vi "Joy Processing.vi"() -> (5 "Plug in titles":string[](array[string]), 7 "Plug in values":string[](array[string]))   [LabVIEW 2021]
uses:
  Globals/Meas_global.vi
panel:
  out "XY Graph":T1(graph)
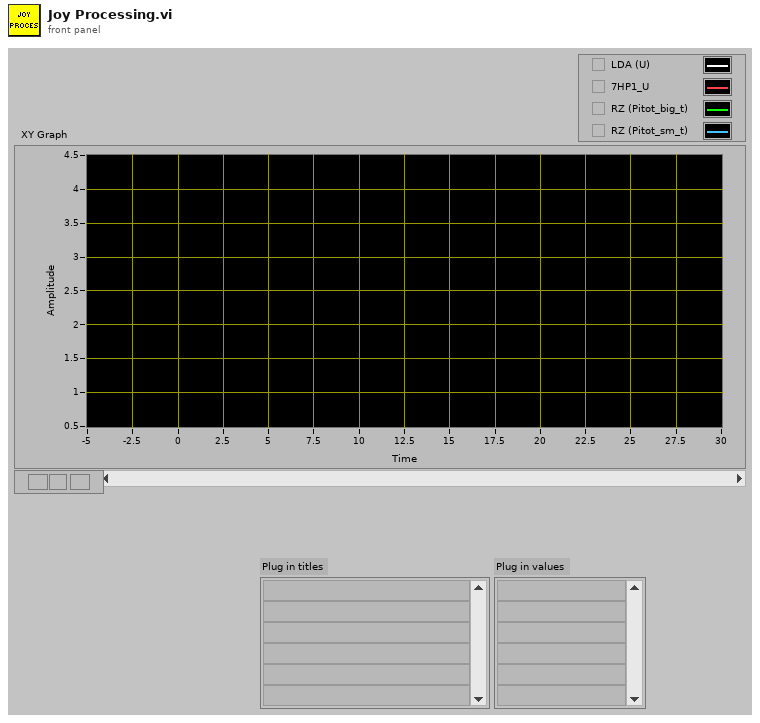
[diagram p1: front panel]
types:
  T1 = cluster{"Time (s)":dbl[], "Velocity (m/s)":dbl[]}[]
  T2 = typedef "Analysis_info_cluster.ctl" = cluster{"Colour":u32, "Inst type":T3, "Inst name":string, "Symbol":string, "Code name":string, "Extra Info":string, "Inst Array":T4, "Extra Titles":string[], "Extra Values":string[], "U":dbl, "u^2":dbl, "u^3":dbl, "u^4":dbl, "Skew_u":dbl, "Kurt_u":dbl, "Sd Error in Mean":dbl, "% u'/U":dbl, "X":dbl, "Y":dbl, "Z":dbl, "Timescale integral Estimate":dbl, "Sd Error in Variance":dbl, "Calib File":path, "Calib Constants":dbl[], "Output Position":bool, "Stats":enum16{"None", "Basic", "Full"}, "Av Sampling Rate":dbl, "Av No of Samples":dbl, "Total Meas Time (s)":dbl, "ADAM Ch Name":string, "Max value":dbl, "Min value":dbl, "Req Sample Rate Hz":dbl, "Sync Delay Time (s)":dbl, "Ch No":i16, "Device":string, "Use Latest Calib":bool, "Port":string, "Metadata Ch Names":string[], "Metadata Ch Values":string[], "Label":string}
  T3 = typedef "Inst_type.ctl" = enum16{"Raw voltage", "Raw with zero offsetting", "Propeller anemometer", "Pressure Transducer", "Pitot-static tube", "Hot wire", "Cross wire 1", "Cross wire 2", "Generic Linear", "Generic Polynomial", "Generic BackPoly", "Fast FID", "Thermocouple", "Cold wire", "Pulsed Wire", "LDA Vel", "LDA Tran time", "LDA Arr time", "Microphone"}
  T4 = typedef "Instrument_Array.ctl" = enum16{"PWA", "LDA", "Analogue"}
  T5 = typedef "Time_Trace_Cluster.ctl" = cluster{"Weighting":dbl[], "Voltage":dbl[], "Eng Values":dbl[]}
  T6 = cluster{"Time (s)":dbl[], "Velocity (m/s)":dbl[]}
  T7 = typedef "Correlation_cluster1.ctl" = cluster{"U inst":string, "uw":dbl, "u^2w":dbl, "uw^2":dbl, "uw/u'w'":dbl, "W inst":string, "uw^3":dbl, "u^3w":dbl, "u^2w^2":dbl, "Index U":i32, "Index W":i32, "Error info":string[], "Paired Sampling Rate (Hz)":dbl, "u^2 Paired":dbl, "w^2 Paired":dbl, "Time Window (ms)":dbl}
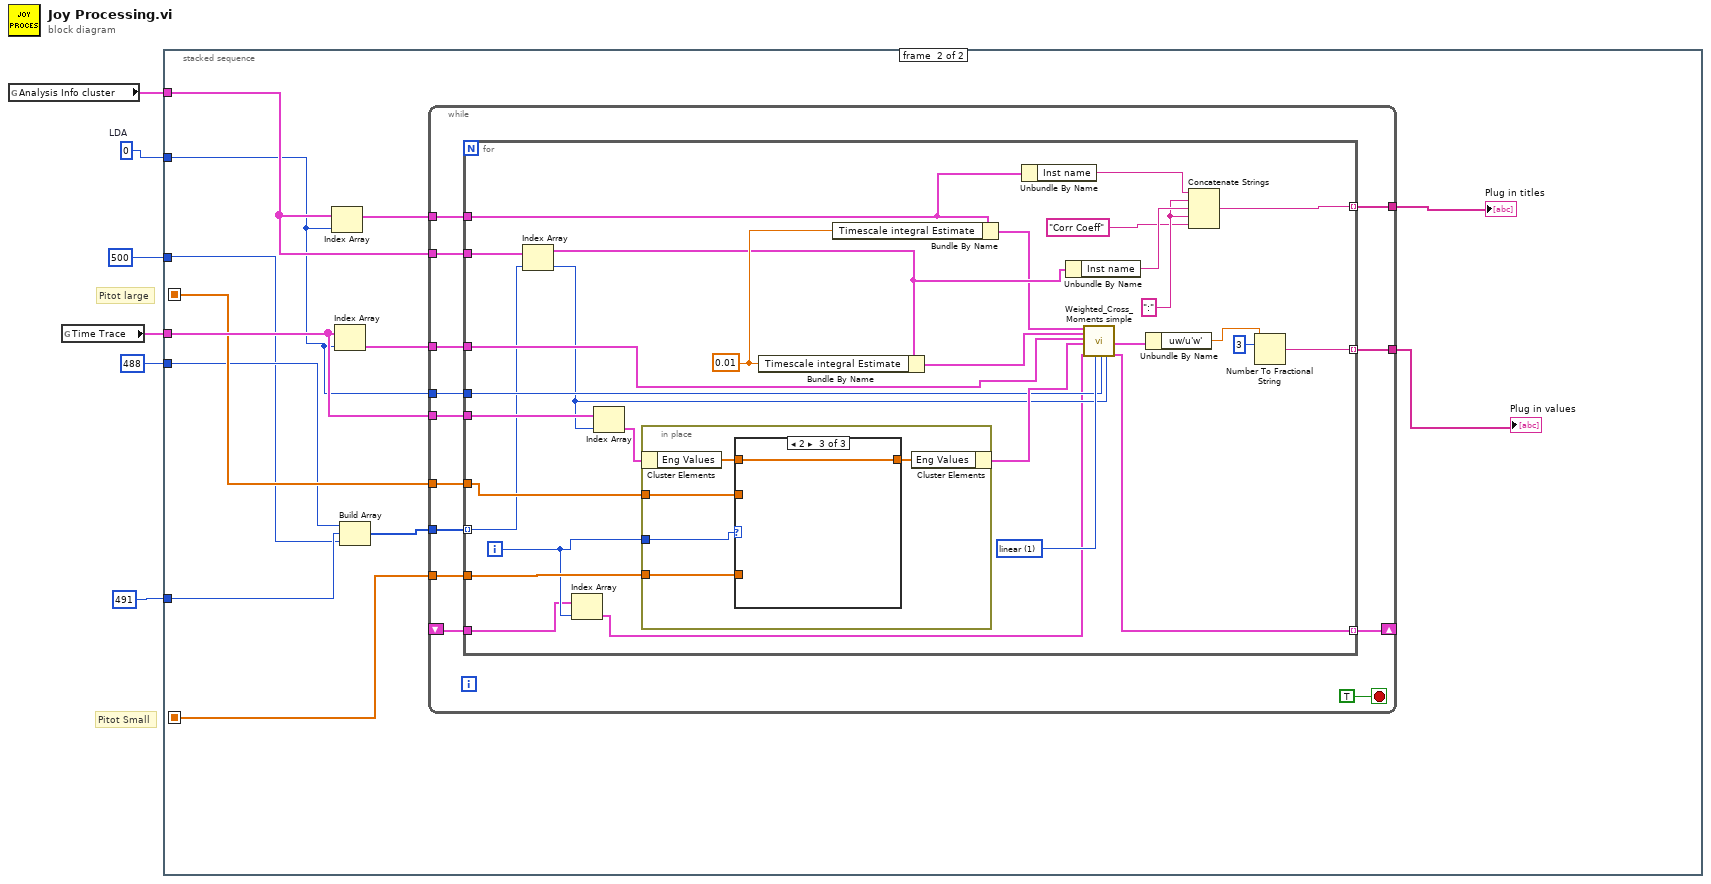
[diagram p0: block diagram]
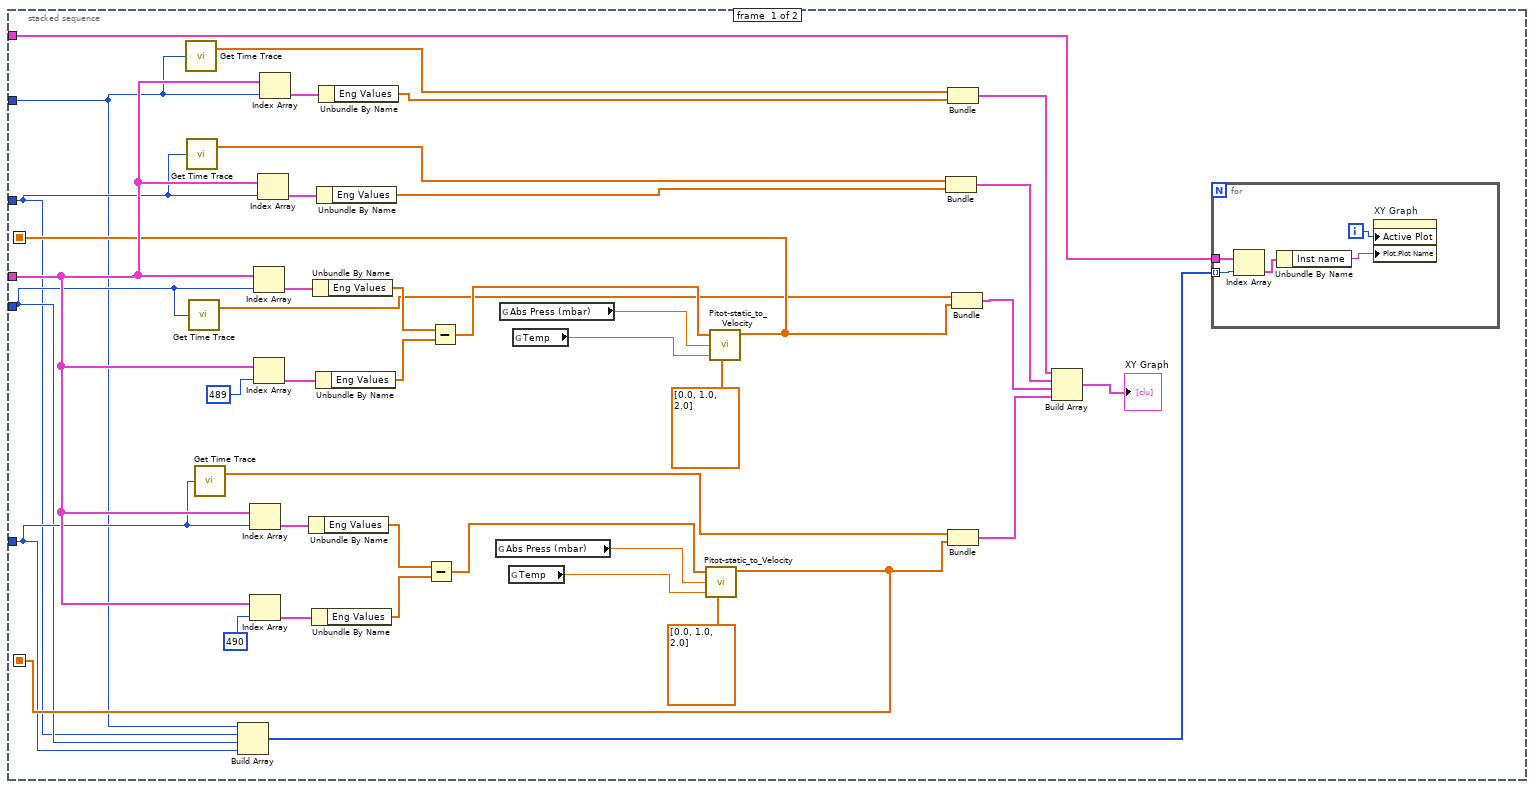
[diagram p2: hidden frame]
diagram:
  w6 = 0  # LDA
  # "Pitot Small"
  # "Pitot large"
  n1 = global read "Meas_global.vi" "Analysis Info cluster"() -> (w2:T2[])
  n2 = global read "Meas_global.vi" "Time Trace"() -> (w5:T5[])
  n3 = stacked-sequence {
    seq-local: [w17 _] -> [_ w61]
    seq-local: [w16 _] -> [_ w56]
    tunnel: w6 -> [w11 w52]
    tunnel: w5 -> [w18 w63]
    tunnel: 488 ("index") -> [w13 w59]
    tunnel: 491 ("index") -> [w14 w58]
    tunnel: w2 -> [w15 w64]
    tunnel: 500 ("index") -> [w12 w53]
    frame #0 {
      n4 = call "Get Time Trace.vi"("Channel Index"=w11) -> ("Time (s)"=w10:dbl[])  [unwired: 1 out]
      n5 = call "Get Time Trace.vi"("Channel Index"=w12) -> ("Time (s)"=w9:dbl[])  [unwired: 1 out]
      n6 = call "Get Time Trace.vi"("Channel Index"=w13) -> ("Time (s)"=w8:dbl[])  [unwired: 1 out]
      n7 = call "Get Time Trace.vi"("Channel Index"=w14) -> ("Time (s)"=w7:dbl[])  [unwired: 1 out]
      n8 = Build Array(w11, w12, w13, w14) -> (w19:i32[])
      n9 = Index Array(array=w18, index=w14) -> (element=w29:T5)
      n10 = Index Array(array=w18, index=490) -> (element=w31:T5)
      n11 = Index Array(array=w18, index=w13) -> (element=w46:T5)
      n12 = Index Array(array=w18, index=489) -> (element=w44:T5)
      n13 = Index Array(array=w18, index=w12) -> (element=w25:T5)
      n14 = Index Array(array=w18, index=w11) -> (element=w21:T5)
      n15 = Unbundle By Name(w29) -> ("Eng Values"=w32:dbl[])
      n16 = Unbundle By Name(w31) -> ("Eng Values"=w33:dbl[])
      n17 = Unbundle By Name(w46) -> ("Eng Values"=w43:dbl[])
      n18 = Unbundle By Name(w44) -> ("Eng Values"=w42:dbl[])
      n19 = Unbundle By Name(w25) -> ("Eng Values"=w24:dbl[])
      n20 = Unbundle By Name(w21) -> ("Eng Values"=w22:dbl[])
      n21 = Subtract(x=w32, y=w33) -> (x-y=w37:dbl[])
      n22 = Subtract(x=w43, y=w42) -> (x-y=w38:dbl[])
      n23 = global read "Meas_global.vi" "Abs Press (mbar)"() -> (w35:dbl)
      n24 = global read "Meas_global.vi" "Abs Press (mbar)"() -> (w40:dbl)
      n25 = global read "Meas_global.vi" "Temp"() -> (w34:dbl)
      n26 = global read "Meas_global.vi" "Temp"() -> (w41:dbl)
      n27 = call "Pitot-static_to_Velocity.vi"("Pressure Trans voltage"=w37, "Atmos Press mbar  (1000)"=w35, "Temp  C  (20)"=w34, "Pressure Trans Calib const"=dbl[] [0.0, 1.0, 2.0]) -> ("Velocity (m/s)"=w16:dbl[])  [unwired: 2 in, 2 out]
      n28 = call "Pitot-static_to_Velocity.vi"("Pressure Trans voltage"=w38, "Atmos Press mbar  (1000)"=w40, "Temp  C  (20)"=w41, "Pressure Trans Calib const"=dbl[] [0.0, 1.0, 2.0]) -> ("Velocity (m/s)"=w17:dbl[])  [unwired: 2 in, 2 out]
      n29 = Bundle("Time (s)"=w9, "Eng Values"=w24) -> (w23:cluster{"Time (s)":dbl[], "Eng Values":dbl[]})  [unwired: 1 in]
      n30 = Bundle("Time (s)"=w10, "Eng Values"=w22) -> (w20:cluster{"Time (s)":dbl[], "Eng Values":dbl[]})  [unwired: 1 in]
      n31 = Bundle("Time (s)"=w7, "Velocity (m/s)"=w16) -> (w28:T6)  [unwired: 1 in]
      n32 = Bundle("Time (s)"=w8, "Velocity (m/s)"=w17) -> (w27:T6)  [unwired: 1 in]
      n33 = Build Array(w20, w23, w27, w28) -> (→"XY Graph":T1)
      n34 = for {
        tunnel: w19 -> [w50] mode=indexing
        tunnel: w15 -> [w47]
        i -> [w51]
        n35 = Index Array(array=w47, index=w50) -> (element=w49:T2)
        n36 = Unbundle By Name(w49) -> ("Inst name"=w48:string)
        n37 = property on="XY Graph" class="XYGraph (strict)"("Active Plot"=w51, "Plot.Plot Name"=w48) -> ()  [unwired: 2 in, 2 out]
      }
    }
    frame #1 {
      n38 = Index Array(array=w64, index=w52) -> (element=w62:T2)
      n39 = Index Array(array=w63, index=w52) -> (element=w60:T5)
      n40 = Build Array(w59, w58, w53) -> (w57:i32[])
      n41 = while {
        tunnel: w64 -> [w77]
        tunnel: w63 -> [w76]
        tunnel: w62 -> [w75]
        tunnel: w61 -> [w74]
        tunnel: w60 -> [w73]
        tunnel: w57 -> [w72]
        tunnel: w56 -> [w71]
        tunnel: [w70] -> w55
        tunnel: [w69] -> w54
        shift-right: [w68] -> _
        shift-left: _ -> [w67]
        tunnel: w52 -> [w66]
        stop <- TRUE stop-if-true
        n42 = for {
          tunnel: w77 -> [w104]
          tunnel: w76 -> [w92]
          tunnel: w75 -> [w99]
          tunnel: w74 -> [w91]
          tunnel: w73 -> [w88]
          tunnel: w72 -> [w81] mode=indexing
          tunnel: w71 -> [w101]
          tunnel: [w100] -> w70 mode=indexing
          tunnel: [w93] -> w69 mode=indexing
          tunnel: [w86] -> w68 mode=indexing
          tunnel: w67 -> [w79]
          tunnel: w66 -> [w82]
          i -> [w80]
          w95 = ":" ("string")
          w103 = 0.01 ("Timescale integral Estimate")
          w85 = 1 items=["nearest", "linear", "spline", "cubic Hermite", "Lagrange"] ("interp. method")
          n43 = Index Array(array=w104, index=w81) -> (element=w98:T2)
          n44 = Index Array(array=w79, index=w80) -> (element=w78:cluster{"Stats":dbl[]})
          n45 = Index Array(array=w92, index=w81) -> (element=w102:T5)
          n46 = in-place {
            in-place-border: w101 -> [w107]
            in-place-border: w80 -> [w110]
            in-place-border: w91 -> [w108]
            n47 = in-place-cluster #1(w102) -> ("Eng Values"=w106:dbl[])
            n48 = case shown="2" w110 {
              tunnel: [w111 w112 w113] -> w109
              tunnel: w108 -> [w111 _ _]
              tunnel: w107 -> [_ w112 _]
              tunnel: w106 -> [_ _ w113]
              frame 0, Default {
              }
              frame 1 {
              }
              frame 2 {
              }
            }
            n49 = in-place-cluster #1("Eng Values"=w109) -> (w87:T5)
          }
          n50 = Bundle By Name(cluster=w98, "Timescale integral Estimate"=w103) -> (w89:T2)
          n51 = Bundle By Name(cluster=w99, "Timescale integral Estimate"=w103) -> (w90:T2)
          n52 = Unbundle By Name(w99) -> ("Inst name"=w97:string)
          n53 = Unbundle By Name(w98) -> ("Inst name"=w96:string)
          n54 = call "Weighted_Cross_Moments simple.vi"("AI Cluster 1"=w90, "AI Cluster 2"=w89, "Time Cluster 1"=w88, "Time Cluster 2"=w87, "Shift Cluster In"=w78, "interp. method"=w85, "Index1"=w82, "Index2"=w81) -> ("output cluster"=w84:T7, "Shift Cluster Out"=w86:cluster{"Stats":dbl[]})  [unwired: 10 in]
          n55 = Unbundle By Name(w84) -> ("uw/u'w'"=w83:dbl)
          n56 = Concatenate Strings(w97, w95, w96, w95, "Corr Coeff" ("string")) -> (w93:string)
          n57 = Number To Fractional String(number=w83, precision (6)=i16 3) -> (F-format string=w100:string)  [unwired: 2 in]
        }
      }
      "Plug in values" <- w55
      "Plug in titles" <- w54
    }
  }
